vi "calc_cycle_length.vi"(0 "burst period":dbl, 2 "burst amount":i32, 5 "mol delay":dbl) -> (7 "exp cycle duration":dbl)   [LabVIEW 2011]
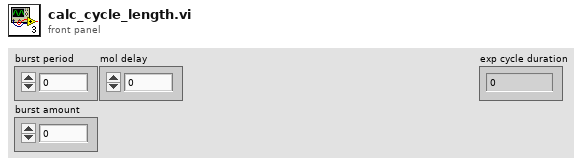
[diagram p1: front panel]
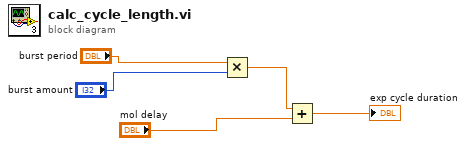
[diagram p0: block diagram]
diagram:
  n1 = Multiply(x="burst period", y="burst amount") -> (x*y=w5:dbl)
  n2 = Add(x=w5, y="mol delay") -> (x+y=→"exp cycle duration":dbl)
